vi "Memory.Pointer.Segment.vi"(7 "segment size":u64 format="%d bytes", 8 "error in (no error)":errorcluster, 9 "count":u64, 10 "segmented pointer type":refnum<class "Memory.Pointer.lvclass">, 11 "base pointer in":refnum<class "Memory.Pointer.lvclass">) -> (0 "error out":errorcluster, 2 "segmented Pointers":refnum<class "Memory.Pointer.lvclass">[](array[class]), 3 "base pointer out":refnum<class "Memory.Pointer.lvclass">)   [LabVIEW 2016, in "Memory.lvlib" / "Memory.Pointer.lvclass"]
uses:
  Memory.Pointer.lvclass
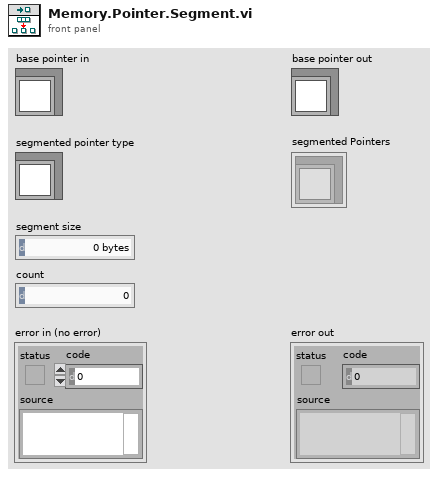
[diagram p1: front panel]
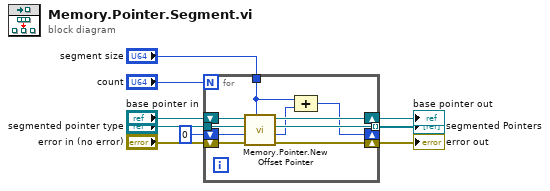
[diagram p0: block diagram]
diagram:
  n1 = for {
    N: "count" -> [_]
    tunnel: "segmented pointer type" -> [w18]
    tunnel: "segment size" -> [w10]
    shift-right: [w17] -> w4
    shift-left: "error in (no error)" -> [w16]
    shift-right: [w15] -> w3
    shift-left: "base pointer in" -> [w19]
    tunnel: [w14] -> w2 mode=indexing
    shift-right: [w11] -> _
    shift-left: u64 0 ("offset (0)") -> [w13]
    n2 = call "Memory.Pointer.New Offset Pointer.vi"("length (-1: rest)"=w10, "error in (no error)"=w16, "offset (0)"=w13, "offset pointer type"=w18, "base pointer in"=w19) -> ("error out"=w17:errorcluster, "offset out"=w12:u64, "offset pointer"=w14:refnum<class "Memory.Pointer.lvclass">, "base pointer out"=w15:refnum<class "Memory.Pointer.lvclass">)  [unwired: 3 in]
    n3 = Compound Arithmetic op=ADD(w10, w12) -> (w11:u64)
  }
  "error out" <- w4
  "base pointer out" <- w3
  "segmented Pointers" <- w2
